vi "Core Action.vi"(8 "error in (no error)":errorcluster, 10 "SECS-II Class In":refnum<class "SECS-II Class.lvclass">, 11 "Scenarios Class in":refnum<class "Scenarios Class.lvclass">) -> (0 "error out":errorcluster, 2 "SECS-II Class Out":refnum<class "SECS-II Class.lvclass">, 3 "Scenarios Class out":refnum<class "Scenarios Class.lvclass">)   [LabVIEW 2020, in "SECS Scenarios.lvlib" / "Scenarios Class.lvclass"]
uses:
  Scenarios Class.lvclass
  SECS Communication/SECS-II Class/SECS-II Class.lvclass
  Reply State.ctl
  Scenarios Class.lvclass/Scenarios Class.ctl
  SECS Communication/SECS-II Class/SECS-II Class.lvclass/SECS-II Class.ctl
  Write Reply State.vi
  SECS Communication/SECS-II Class/Read W-Bit.vi
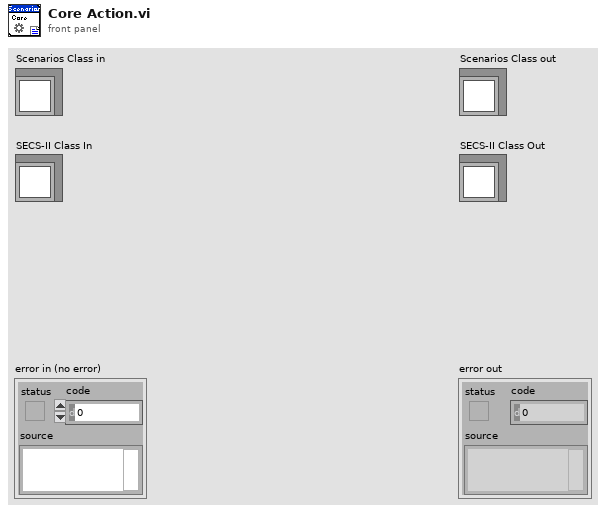
[diagram p1: front panel]
types:
  T1 = typedef "SECS Scenarios.lvlib/Scenarios Class.lvclass/Reply State.ctl" = enum16{"OK", "Illegal Data", "Unknown Stream", "Unknown Function", "Off-Line", "T3 Timeout", "Inner-Timeout"}
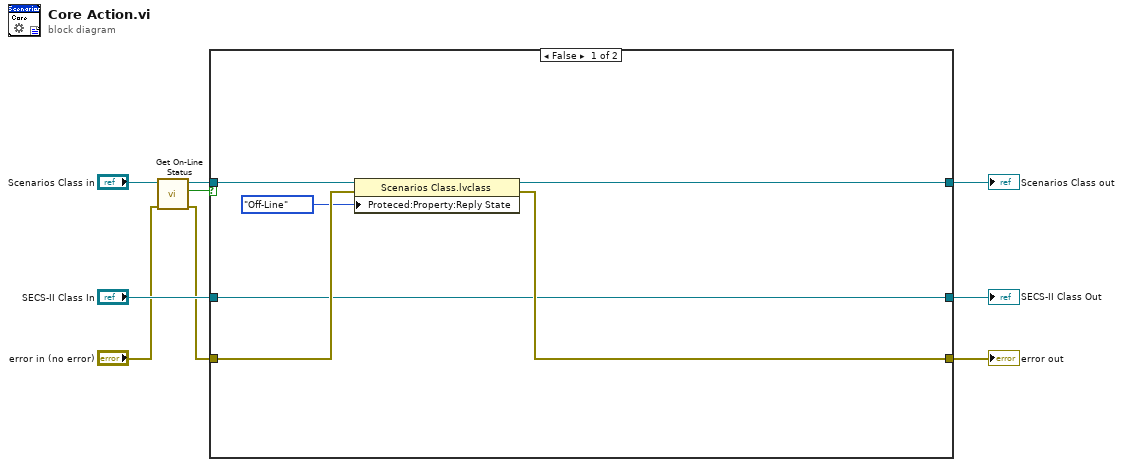
[diagram p0: block diagram]
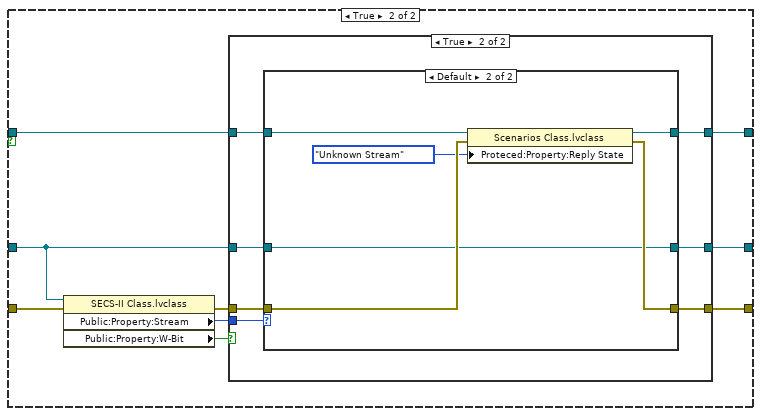
[diagram p2: hidden frame]
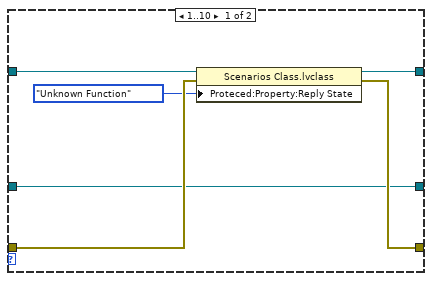
[diagram p4: hidden frame]
diagram:
  n1 = call "Get On-Line Status.vi"("error in (no error)"="error in (no error)", "Scenarios Class in"="Scenarios Class in") -> ("error out"=w3:errorcluster, "On-Line"=w2:bool, "Scenarios Class out"=w4:refnum<class "Scenarios Class.lvclass">)  [unwired: 7 in]
  n2 = case shown="False" w2 {
    tunnel: [w13 w22] -> w9
    tunnel: [w12 w21] -> w8
    tunnel: "SECS-II Class In" -> [w11 w20]
    tunnel: [w11 w19] -> w6
    tunnel: w4 -> [w14 w17]
    tunnel: w3 -> [w15 w16]
    frame False {
      n3 = property class="Scenarios Class.lvclass"(reference=w14, error in=w15, "Proteced:Property:Reply State"=Reply_State."Off-Line" ("Reply State")) -> (reference out=w13:refnum<class "Scenarios Class.lvclass">, error out=w12:errorcluster)
    }
    frame True {
      n4 = property class="SECS-II Class.lvclass"(reference=w20, error in=w16) -> (error out=w24:errorcluster, "Public:Property:Stream"=w23:u8, "Public:Property:W-Bit"=w18:bool)  [unwired: 1 out]
      n5 = case shown="True" w18 {
        tunnel: w24 -> [w25 w34]
        tunnel: w23 -> [_ w33]
        tunnel: w17 -> [w27 w32]
        tunnel: [w27 w31] -> w22
        tunnel: [w25 w30] -> w21
        tunnel: w20 -> [w26 w29]
        tunnel: [w26 w28] -> w19
        frame False {
        }
        frame True {
          n6 = case shown="Default" w33 {
            tunnel: w34 -> [w38 w44]
            tunnel: [w37 w43] -> w30
            tunnel: w32 -> [w40 w46]
            tunnel: [w39 w45] -> w31
            tunnel: w29 -> [w36 w42]
            tunnel: [w36 w42] -> w28
            frame 1..10 {
              # "Unknown Function"
              n7 = property class="Scenarios Class.lvclass"(reference=w40, error in=w38, "Proteced:Property:Reply State"=Reply_State."Unknown Function" ("Reply State")) -> (reference out=w39:refnum<class "Scenarios Class.lvclass">, error out=w37:errorcluster)
            }
            frame Default {
              # "Unknown Function"
              n8 = property class="Scenarios Class.lvclass"(reference=w46, error in=w44, "Proteced:Property:Reply State"=Reply_State."Unknown Stream" ("Reply State")) -> (reference out=w45:refnum<class "Scenarios Class.lvclass">, error out=w43:errorcluster)
            }
          }
        }
      }
    }
  }
  "error out" <- w8
  "Scenarios Class out" <- w9
  "SECS-II Class Out" <- w6
